vi "UIDisableyesno.vi"(8 "error in (no error)":errorcluster, 10 "UI":T1, 11 "Status:":refnum<vi>) -> (0 "error out":errorcluster)   [LabVIEW 2021]
uses:
  Global Variablesyes.vi
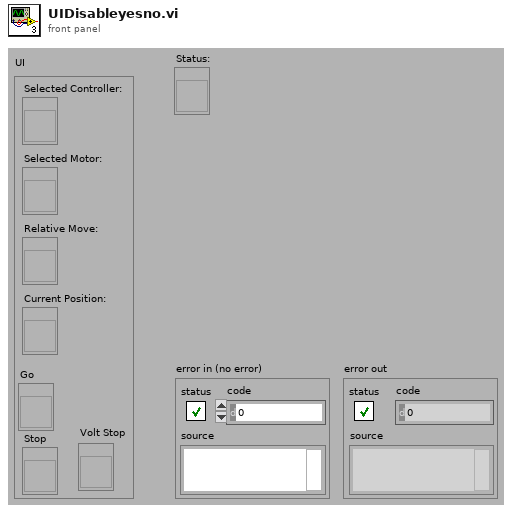
[diagram p1: front panel]
types:
  T1 = cluster{"Selected Controller:":refnum<vi>, "Selected Motor:":refnum<vi>, "Relative Move:":refnum<vi>, "Current Position:":refnum<vi>, "Go":refnum<vi>, "Stop":refnum<vi>, "Volt Stop":refnum<vi>}
  T2 = enum8{"Enabled", "Disabled", "Disabled and Grayed Out"}
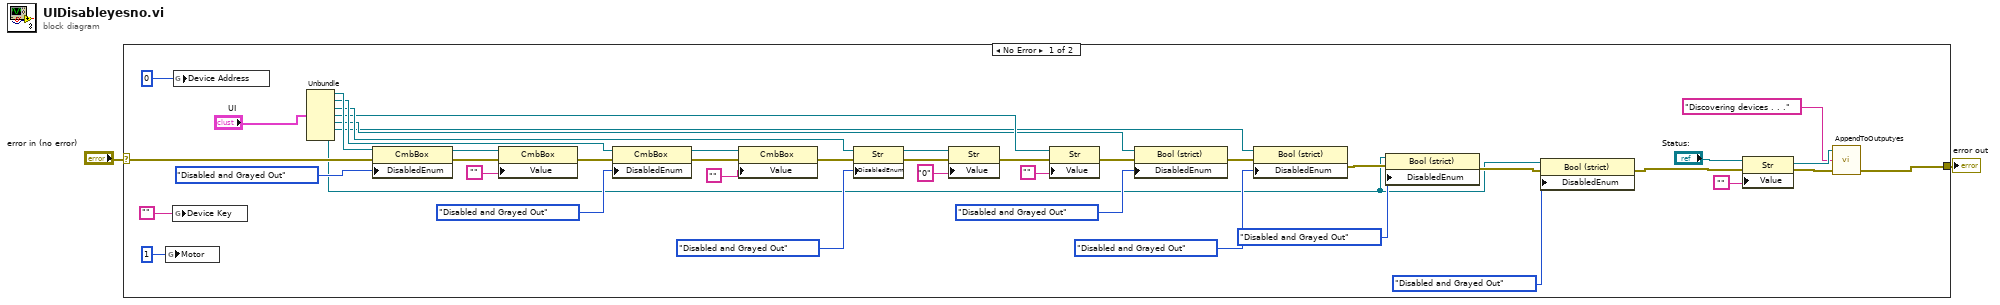
[diagram p0: block diagram]
diagram:
  n1 = case shown="No Error" "error in (no error)" {
    selector: "error in (no error)" -> [w38 w46]
    tunnel: [w28 w46] -> w1
    frame No Error {
      n2 = global write "Global Variablesyes.vi" "Motor"(1 ("Motor")) -> ()
      n3 = global write "Global Variablesyes.vi" "Device Key"("") -> ()
      n4 = global write "Global Variablesyes.vi" "Device Address"(0 ("Device Address")) -> ()
      n5 = Unbundle("UI") -> ("Selected Controller:"=w14:refnum<vi>, "Selected Motor:"=w13:refnum<vi>, "Relative Move:"=w12:refnum<vi>, "Current Position:"=w11:refnum<vi>, "Go"=w10:refnum<vi>, "Stop"=w9:refnum<vi>, "Volt Stop"=w3:refnum<vi>)
      n6 = property on="Property Node" class="CmbBox"(reference=w14, error in=w38, "DisabledEnum"=T2."Disabled and Grayed Out" ("Disabled")) -> (reference out=w37:refnum<vi>, error out=w33:errorcluster)
      n7 = property class="CmbBox"(reference=w37, error in=w33, "Value"="") -> (error out=w32:errorcluster)  [unwired: 1 out]
      n8 = property on="Property Node" class="CmbBox"(reference=w13, error in=w32, "DisabledEnum"=T2."Disabled and Grayed Out" ("Disabled")) -> (reference out=w35:refnum<vi>, error out=w31:errorcluster)
      n9 = property class="CmbBox"(reference=w35, error in=w31, "Value"="") -> (error out=w30:errorcluster)  [unwired: 1 out]
      n10 = property on="Property Node" class="Str"(reference=w12, error in=w30, "DisabledEnum"=T2."Disabled and Grayed Out" ("Disabled")) -> (reference out=w22:refnum<vi>, error out=w23:errorcluster)
      n11 = property class="Str"(reference=w22, error in=w23, "Value"="0") -> (error out=w20:errorcluster)  [unwired: 1 out]
      n12 = property on="Property Node" class="Str"(reference=w11, error in=w20, "Value"="") -> (error out=w19:errorcluster)  [unwired: 1 out]
      n13 = property on="Property Node" class="Bool (strict)"(reference=w10, error in=w19, "DisabledEnum"=T2."Disabled and Grayed Out" ("Disabled")) -> (error out=w40:errorcluster)  [unwired: 1 out]
      n14 = property on="Property Node" class="Bool (strict)"(reference=w9, error in=w40, "DisabledEnum"=T2."Disabled and Grayed Out" ("Disabled")) -> (error out=w7:errorcluster)  [unwired: 1 out]
      n15 = property on="Property Node" class="Bool (strict)"(reference=w3, error in=w7, "DisabledEnum"=T2."Disabled and Grayed Out" ("Disabled")) -> (error out=w5:errorcluster)  [unwired: 1 out]
      n16 = property on="Property Node" class="Bool (strict)"(reference=w3, error in=w5, "DisabledEnum"=T2."Disabled and Grayed Out" ("Disabled")) -> (error out=w4:errorcluster)  [unwired: 1 out]
      n17 = property class="Str"(reference="Status:", error in=w4, "Value"="") -> (reference out=w29:refnum<vi>, error out=w27:errorcluster)
      n18 = call "AppendToOutputyes.vi"("error in"=w27, "Input String"="Discovering devices . . .", "Output Refnum In"=w29) -> ("error out"=w28:errorcluster)  [unwired: 1 in, 1 out]
    }
    frame Error {
    }
  }
  "error out" <- w1
